vi "QueryServer_GetRequest_Query.vi"(0 "gRPCid":T1, 3 "error in (no error)":errorcluster) -> (7 "gRPCid out":T1, 9 "query":string, 10 "error out":errorcluster)   [LabVIEW 2019, in "labview-grpc-query-server.lvlib"]
uses:
  labview-grpc-query-server.lvlib
  gRPC interface/Server API/typeDefs/grpcId.ctl
  QueryServer_QueryRequest.ctl
  6d6a72de-64f3-4912-b6d0-fc0b84b2ddfc.vi
  gRPC interface/gprc-lvsupport.lvlib
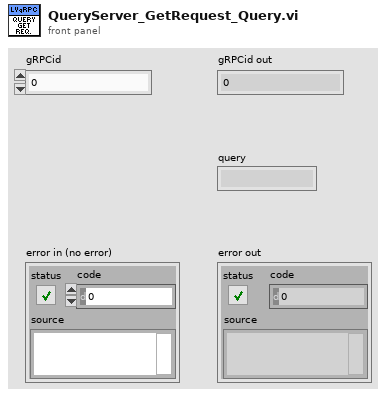
[diagram p1: front panel]
types:
  T1 = typedef "gprc-lvsupport.lvlib/grpcId.ctl" = u64
  T2 = typedef "labview-grpc-query-server.lvlib/QueryServer_QueryRequest.ctl" = cluster{"query":string}
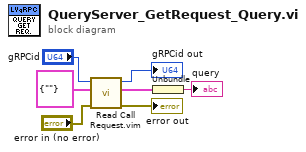
[diagram p0: block diagram]
diagram:
  n1 = call "Read Call Request.vim"("error in (no error)"="error in (no error)", "Data Type"=T2 {"query"=""} ("QueryRequest"), "gRPCid in"="gRPCid") -> ("error out"=→"error out":errorcluster, "Request Data"=w5:T2, "gRPCid out"=→"gRPCid out":T1)  [unwired: 6 in]
  n2 = Unbundle(w5) -> ("query"=→"query":string)
